vi "Set Motor by Label.vi"(8 "error in (no error)":errorcluster, 10 "Motor obj":refnum<class "Motor.lvclass">, 11 "MotionSystem in":refnum<class "MotionSystem.lvclass">) -> (0 "error out":errorcluster, 3 "MotionSystem out":refnum<class "MotionSystem.lvclass">)   [LabVIEW 2016, in "MotionSystem.lvlib" / "MotionSystem.lvclass"]
uses:
  <userlib>/Common Components/Hardware/Abstract System/MotionSystem/MotionSystem/MotionSystem.lvclass
  <userlib>/Common Components/Hardware/Motor/Motor/Motor.lvclass
  C:/Program Files (x86)/National Instruments/LabVIEW 2016/user.lib/Common Components/Hardware/Abstract Hardware/Hardware.lvclass
  <userlib>/Common Components/Hardware/Abstract Hardware/Hardware.lvclass/Hardware.ctl
  <userlib>/Common Components/Hardware/Abstract System/MotionSystem/MotionSystem/MotionSystem.lvclass/MotionSystem.ctl
  <userlib>/Common Components/Hardware/Abstract Hardware/Read Label.vi
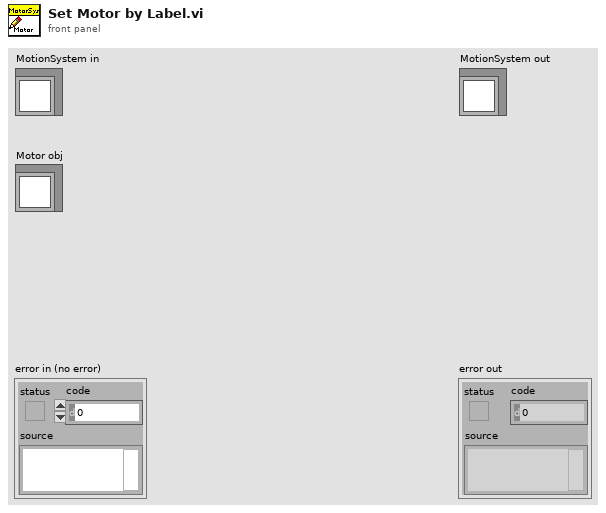
[diagram p1: front panel]
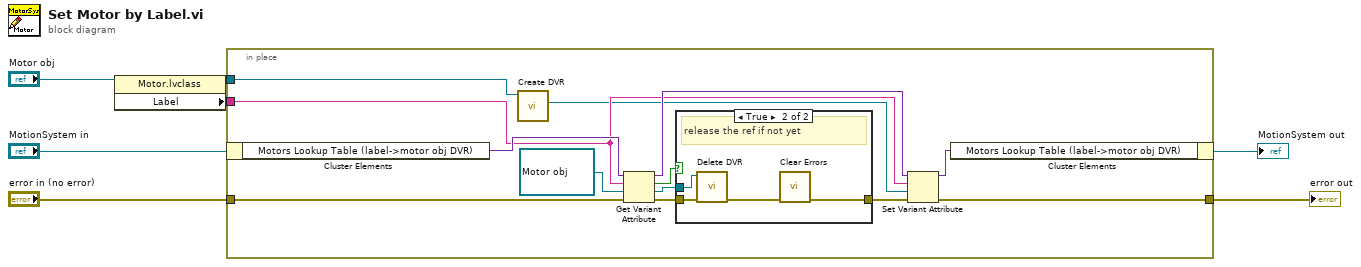
[diagram p0: block diagram]
diagram:
  n1 = property class="Motor.lvclass"(reference="Motor obj") -> (reference out=w4:refnum<class "Motor.lvclass">, "Label"=w3:string)  [unwired: 1 in, 1 out]
  n2 = in-place {
    in-place-border: w4 -> [w18]
    in-place-border: w3 -> [w15]
    in-place-border: "error in (no error)" -> [w11]
    in-place-border: [w20] -> w1
    n3 = in-place-cluster #1("MotionSystem in") -> ("Motors Lookup Table (label->motor obj DVR)"=w17:variant)
    n4 = call <userlib>:"Create DVR.vi"("Motor in"=w18) -> ("data value reference"=w8:refnum<data-value>)  [unwired: 8 in, 2 out]
    n5 = Get Variant Attribute(Variant=w17, name=w15, default value (empty Variant)=refnum<data-value> refnum ("data value reference"), error in=w11) -> (duplicate Variant=w16:variant, found=w13:bool, value=w12:refnum<data-value>, error out=w10:errorcluster)
    n6 = case shown="True" w13 {
      tunnel: w12 -> [_ w25]
      tunnel: w10 -> [w21 w24]
      tunnel: [w21 w22] -> w9
      frame False {
      }
      frame True {
        # "release the ref if not yet"
        n7 = call <userlib>:"Delete DVR.vi"("error in (no error)"=w24, "data value reference"=w25) -> ("error out"=w23:errorcluster)  [unwired: 8 in, 1 out]
        n8 = call <vilib>:"Clear Errors.vi"("error in (no error)"=w23) -> ("error out"=w22:errorcluster)  [unwired: 5 in, 1 out]
      }
    }
    n9 = Set Variant Attribute(Variant=w16, name=w15, value=w8, error in=w9) -> (Variant out=w19:variant, error out=w20:errorcluster)  [unwired: 1 out]
    n10 = in-place-cluster #1("Motors Lookup Table (label->motor obj DVR)"=w19) -> (→"MotionSystem out":refnum<class "MotionSystem.lvclass">)
  }
  "error out" <- w1
